vi "Print Interactions.vi"(8 "error in (no error)":errorcluster, 10 "Interaction Ranges":cluster{"From":dbl, "To":dbl}[](array[cluster]), 11 "Interaction Types":string[](array[string])) -> (0 "error out":errorcluster, 3 "Array":string[](array[string]))   [LabVIEW 2020, in "Topas4.lvlib"]
uses:
  Topas4.lvlib
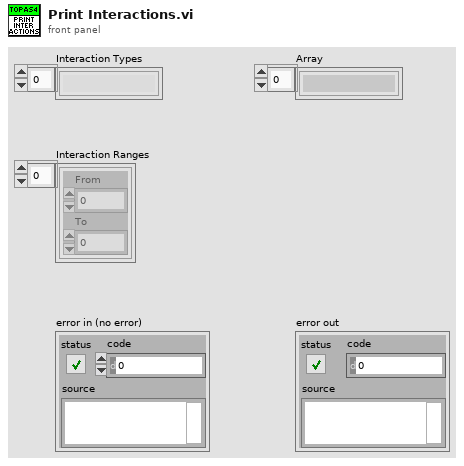
[diagram p1: front panel]
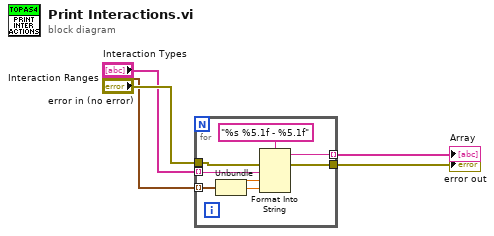
[diagram p0: block diagram]
diagram:
  n1 = for {
    tunnel: "Interaction Ranges" -> [w13] mode=indexing
    tunnel: "Interaction Types" -> [w11] mode=indexing
    tunnel: "error in (no error)" -> [w8]
    tunnel: [w7] -> w4
    tunnel: [w6] -> w5 mode=indexing
    n2 = Unbundle(w13) -> ("From"=w10:dbl, "To"=w9:dbl)
    n3 = Format Into String(format string="%s %5.1f - %5.1f", error in=w8, w11, w10, w9) -> (resulting string=w6:string, error out=w7:errorcluster)  [unwired: 1 in]
  }
  "Array" <- w5
  "error out" <- w4
